vi "matt n' ryan's prime stuff, kittens.vi"() -> ()   [LabVIEW 2012]
panel:
  out "isPrime":bool
  in  "blah":dbl
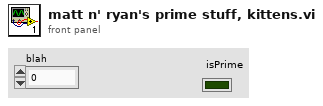
[diagram p1: front panel]
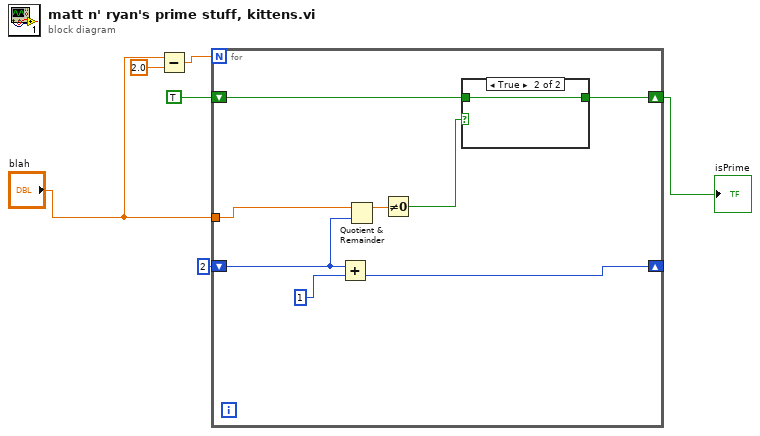
[diagram p0: block diagram]
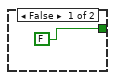
[diagram p2: hidden frame]
diagram:
  n1 = Subtract(x="blah", y=2.0) -> (x-y=w3:dbl)
  n2 = for {
    N: w3 -> [_]
    shift-right: [w12] -> _
    shift-left: 2 -> [w10]
    tunnel: "blah" -> [w14]
    shift-right: [w8] -> w1
    shift-left: TRUE -> [w9]
    n3 = Add(x=w10, y=1) -> (x+y=w12:i32)
    n4 = Quotient & Remainder(x=w14, y=w10) -> (x-y*floor(x/y)=w13:dbl)  [unwired: 1 out]
    n5 = Not Equal To 0?(x=w13) -> (x != 0?=w7:bool)
    n6 = case shown="True" w7 {
      tunnel: w9 -> [_ w16]
      tunnel: [FALSE w16] -> w8
      frame False {
      }
      frame True {
      }
    }
  }
  "isPrime" <- w1
